vi "GetFrame.vi"(8 "error in (no error)":errorcluster, 11 "CameraLan in":refnum<class "CameraLan.lvclass">) -> (0 "error out":errorcluster, 1 "acquired FPS":dbl, 2 "Image Out":T1, 3 "CameraLan out":refnum<class "CameraLan.lvclass">, 4 "status":bool)   [LabVIEW 2011, in "CameraLan.lvclass"]
uses:
  CameraLan.lvclass
  <vilib>/vision/Image Controls.llb/IMAQ Image.ctl
  CameraLan.lvclass/CameraLan.ctl
  <vilib>/vision/driver/NI_Vision_Acquisition_Software.lvlib
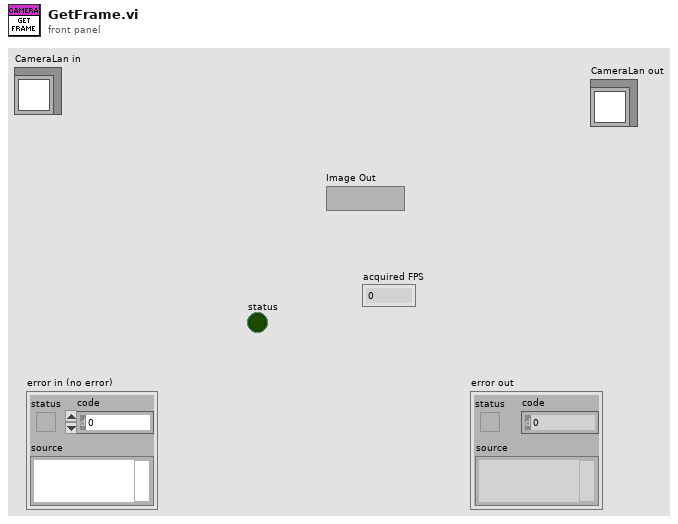
[diagram p1: front panel]
types:
  T1 = typedef "IMAQ Image.ctl" = refnum<image>
  T2 = typedef "IMAQdx.ctl" = refnum<k21>
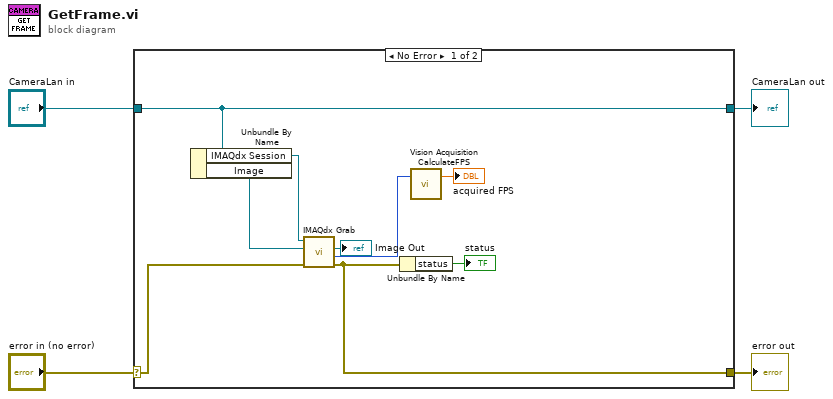
[diagram p0: block diagram]
diagram:
  n1 = case shown="No Error" "error in (no error)" {
    selector: "error in (no error)" -> [w6 w15]
    tunnel: [w5 w15] -> w3
    tunnel: [w12 w14] -> w1
    tunnel: "CameraLan in" -> [w12 w14]
    frame No Error {
      n2 = Unbundle By Name(w12) -> ("IMAQdx Session"=w11:T2, "Image"=w10:T1)
      n3 = call <vilib>:"IMAQdx Grab.vi"("error in"=w6, "Image In"=w10, "Session In"=w11) -> ("error out"=w5:errorcluster, "Buffer Number Out"=w13:u32, "Image Out"=→"Image Out":T1)  [unwired: 1 in, 5 out]
      n4 = Unbundle By Name(w5) -> ("status"=→"status":bool)
      n5 = call <vilib>:"Vision Acquisition CalculateFPS.vi"("buffer number"=w13) -> ("acquired FPS"=→"acquired FPS":dbl)  [unwired: 2 out]
    }
    frame Error {
    }
  }
  "error out" <- w3
  "CameraLan out" <- w1
